vi "MC Read Encoders.vi"(8 "error in (no error)":errorcluster, 10 "Clear Encoders":bool, 11 "VISA resource name":refnum<visa-resource-name>) -> (0 "error out":errorcluster, 1 "Right Encoder Read Dec":u32, 2 "Left Encoder Read Dec":u32)   [LabVIEW 2009]
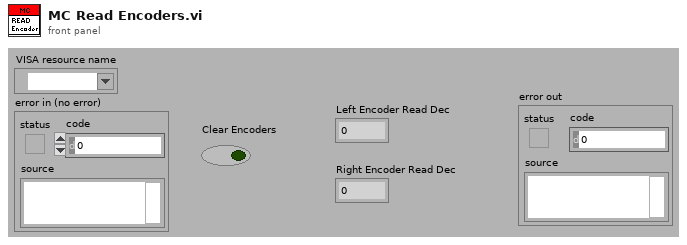
[diagram p1: front panel]
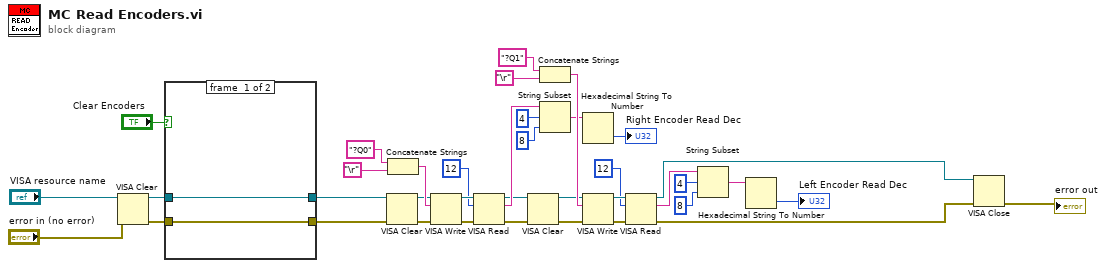
[diagram p0: block diagram]
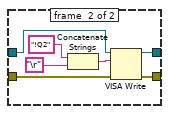
[diagram p2: hidden frame]
diagram:
  n1 = VISA Clear(VISA resource name="VISA resource name", error in (no error)="error in (no error)") -> (VISA resource name out=w37:refnum<visa-resource-name>, error out=w36:errorcluster)
  n2 = case shown="True" "Clear Encoders" {
    tunnel: [w40 w44] -> w35
    tunnel: w37 -> [w40 w47]
    tunnel: [w39 w45] -> w34
    tunnel: w36 -> [w39 w46]
    frame #0 {
    }
    frame #1 {
      n3 = Concatenate Strings("!Q2", "\r") -> (w41:string)
      n4 = VISA Write(VISA resource name=w47, write buffer=w41, error in (no error)=w46) -> (VISA resource name out=w44:refnum<visa-resource-name>, error out=w45:errorcluster)  [unwired: 1 out]
    }
  }
  n5 = VISA Clear(VISA resource name=w35, error in (no error)=w34) -> (VISA resource name out=w25:refnum<visa-resource-name>, error out=w24:errorcluster)
  n6 = Concatenate Strings("?Q0", "\r") -> (w26:string)
  n7 = VISA Write(VISA resource name=w25, write buffer=w26, error in (no error)=w24) -> (VISA resource name out=w30:refnum<visa-resource-name>, error out=w29:errorcluster)  [unwired: 1 out]
  n8 = VISA Read(VISA resource name=w30, byte count=u32 12, error in (no error)=w29) -> (VISA resource name out=w8:refnum<visa-resource-name>, read buffer=w12:string, error out=w7:errorcluster)  [unwired: 1 out]
  n9 = VISA Clear(VISA resource name=w8, error in (no error)=w7) -> (VISA resource name out=w16:refnum<visa-resource-name>, error out=w15:errorcluster)
  n10 = Concatenate Strings("?Q1", "\r") -> (w21:string)
  n11 = String Subset(string=w12, offset (0)=4, length (rest)=u32 8 ("byte count")) -> (substring=w9:string)
  n12 = Hexadecimal String To Number(string=w9) -> (number=→"Right Encoder Read Dec":u32)  [unwired: 2 in, 1 out]
  n13 = VISA Write(VISA resource name=w16, write buffer=w21, error in (no error)=w15) -> (VISA resource name out=w17:refnum<visa-resource-name>, error out=w18:errorcluster)  [unwired: 1 out]
  n14 = VISA Read(VISA resource name=w17, byte count=u32 12, error in (no error)=w18) -> (VISA resource name out=w33:refnum<visa-resource-name>, read buffer=w4:string, error out=w32:errorcluster)  [unwired: 1 out]
  n15 = String Subset(string=w4, offset (0)=4, length (rest)=u32 8 ("byte count")) -> (substring=w3:string)
  n16 = Hexadecimal String To Number(string=w3) -> (number=→"Left Encoder Read Dec":u32)  [unwired: 2 in, 1 out]
  n17 = VISA Close(VISA resource name=w33, error in (no error)=w32) -> (error out=→"error out":errorcluster)
